vi "Main_Power.vi"() -> ()   [LabVIEW 2020]
uses:
  States.ctl
  <vilib>/Instr/_visa.llb/VISA Configure Serial Port (Serial Instr).vi
  <vilib>/Utility/file.llb/Read Delimited Spreadsheet (I64).vi
panel:
  in  "Toggle Power DAQ":bool
  out "Power":dynamicdata(graph)
  out "Last Inc Sent":string
  out "Last Speed Sent":string
  out "Next Control State":T1
  out "Next Com State":enum16{"Initialize", "Send", "Receive", "Error"}(ring)=enum."Receive"
  out "Next Cmd":enum16{"getParm", "inc", "mph", "err"}(ring)
  out "Send Buffer":string
  out "Control Error":errorcluster
  out "Com Error":errorcluster
  out "Missed Msg":u16
  out "Time Left":u32
  out "Inc Changed":bool
  out "Next MPH":u16
  out "Next Duration":u16
  out "Next Inc":u16
  out "PD READ":u8
  out "INC READ":u8
  out "MPH READ":u8
  out "dwell":u16[](array[numeric])
  out "incline":u16[](array[numeric])
  out "time":u16[](array[numeric])
  out "speed":u16[](array[numeric])
  out "input lines":i32
  in  "TestScript":path=path "C:/LabView Computer Backup SEAL2788/DonP_TRM500/FootTimeInc.txt"
  out "read buffer":string
  out "Speed Changed":bool
  in  "Manual Stop":bool
  in  "Serial Port":refnum<visa-resource-name>="COM8"
  out "FootPath":path
  out "FootPathRef":refnum<file>
  out "stopping":bool
  out "Target MPH":u16 max=12 step=1
  out "step":i32
  out "Target INC":u16 max=12 step=1
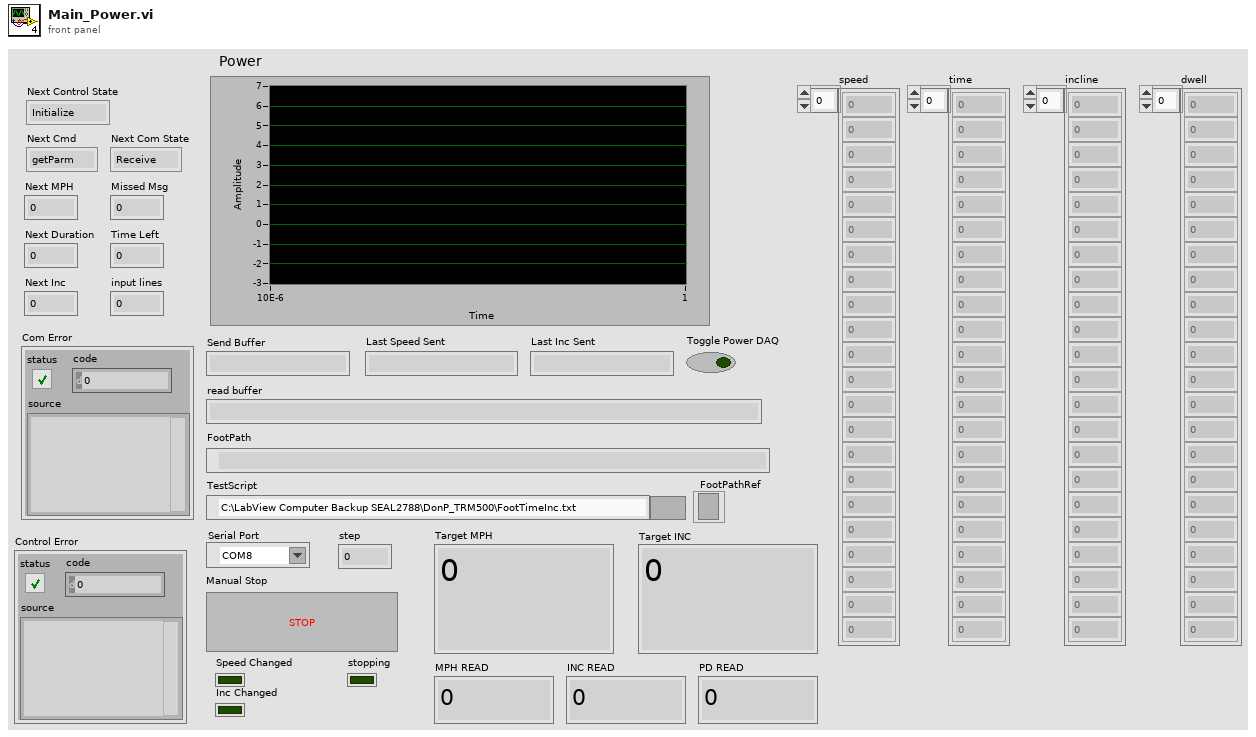
[diagram p1: front panel]
types:
  T1 = typedef "States.ctl" = enum16{"Initialize", "SetTargets", "WaitforMPH", "Dwell", "CheckTiming"}
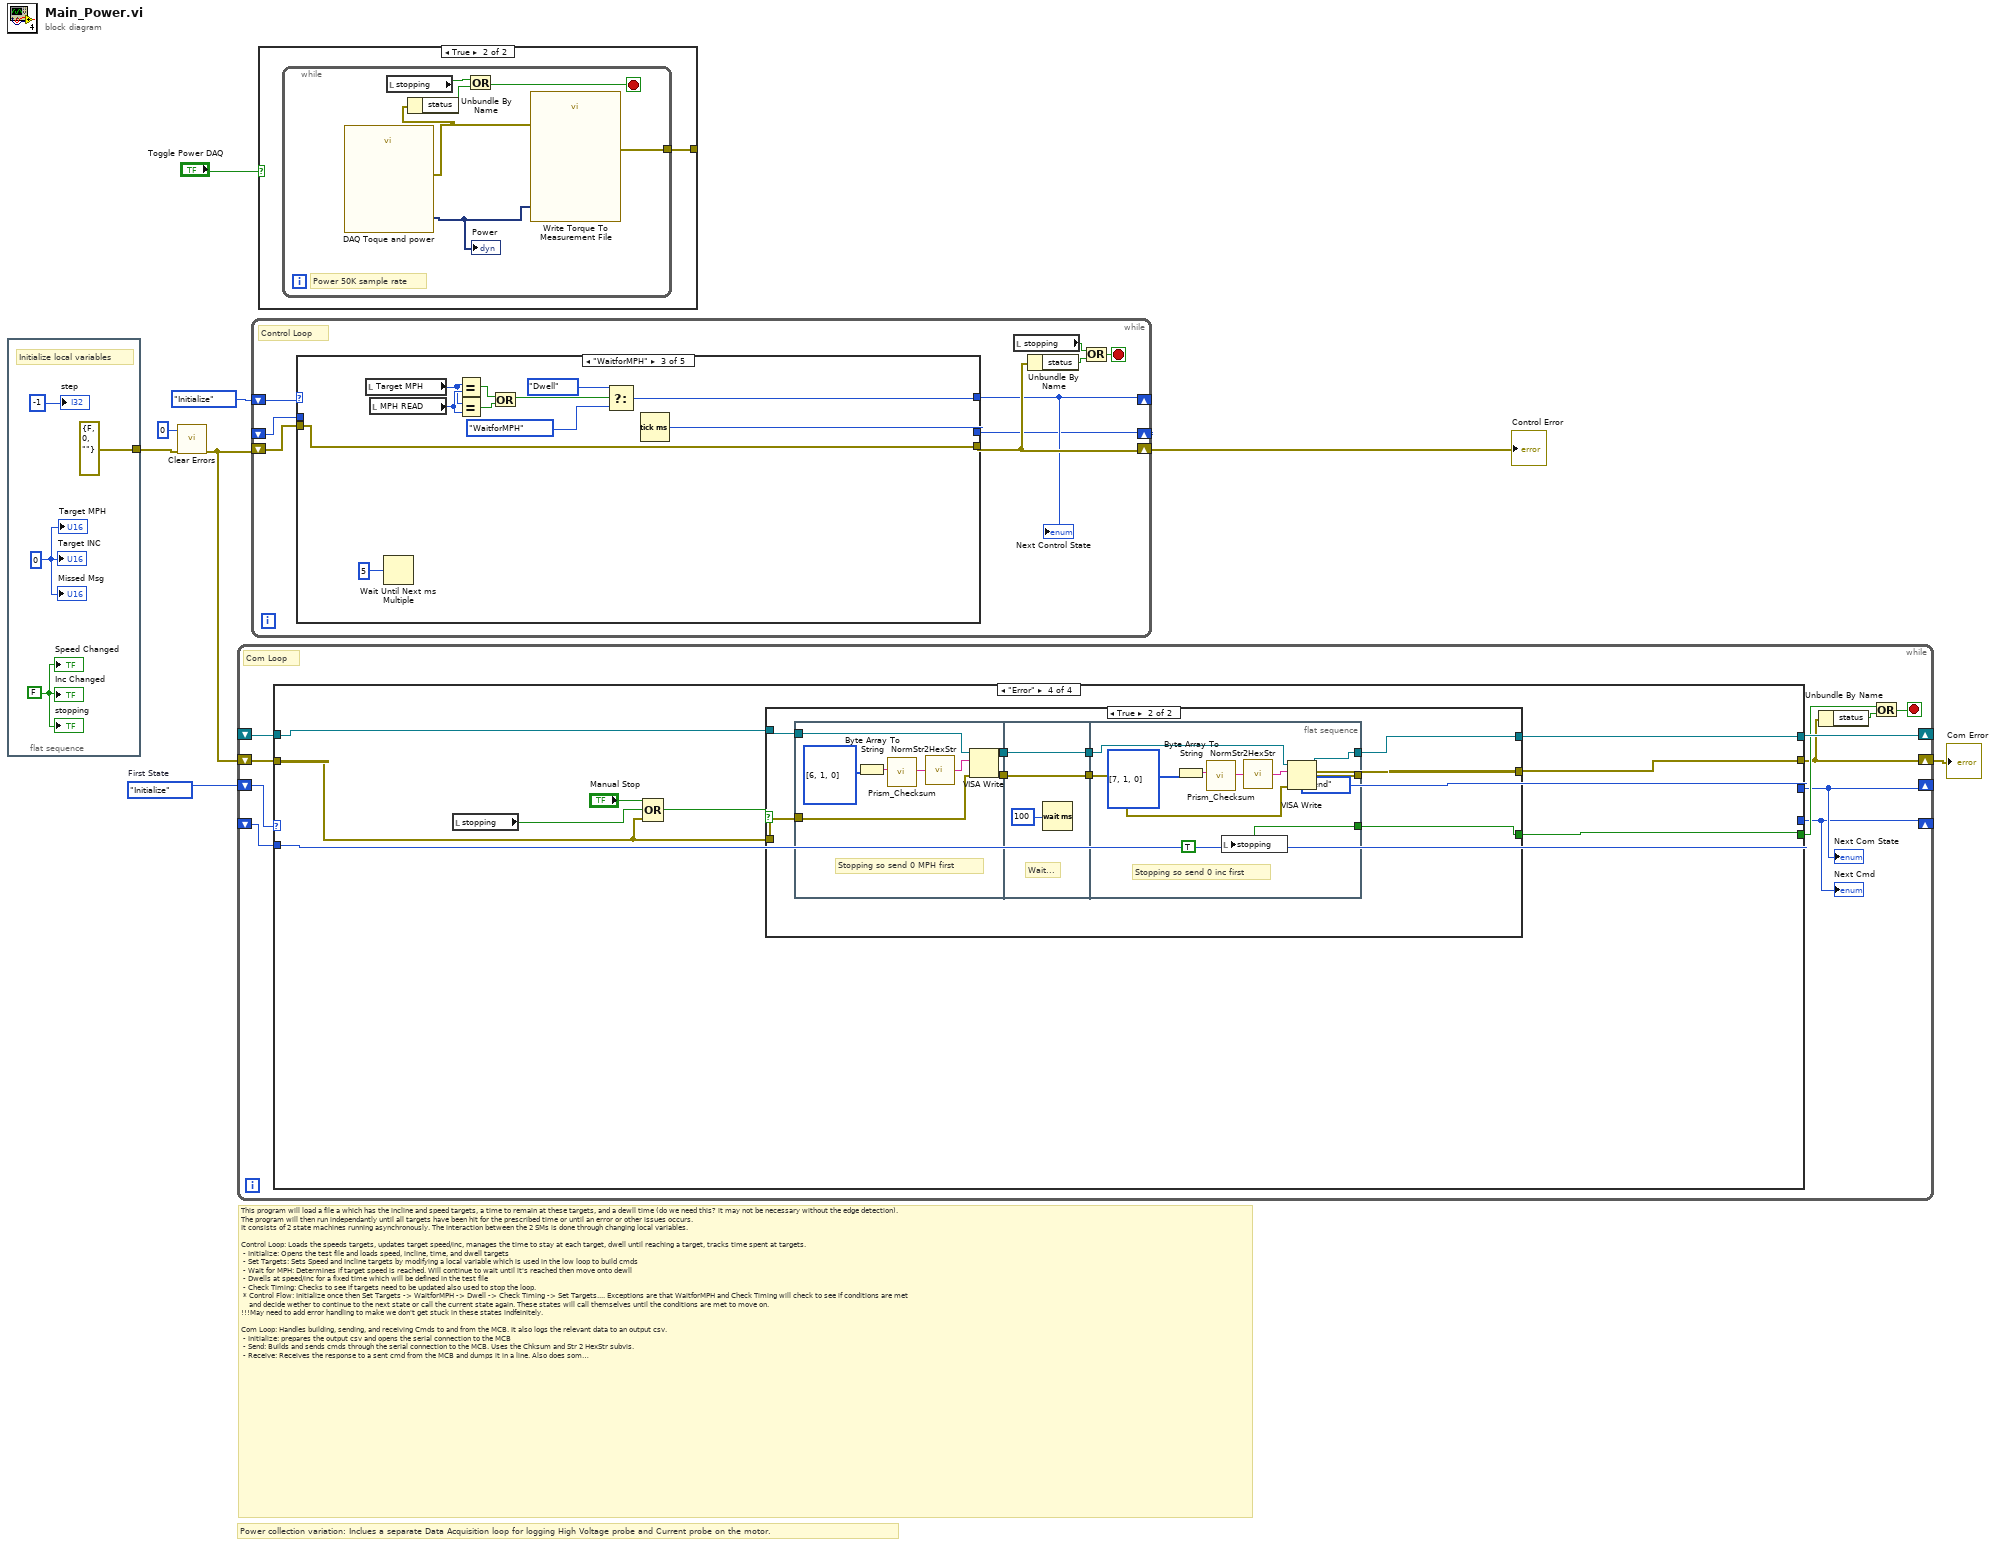
[diagram p0: block diagram]
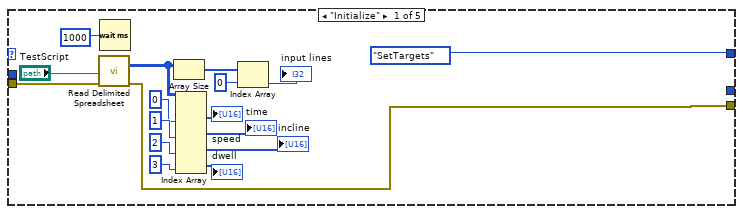
[diagram p3: hidden frame]
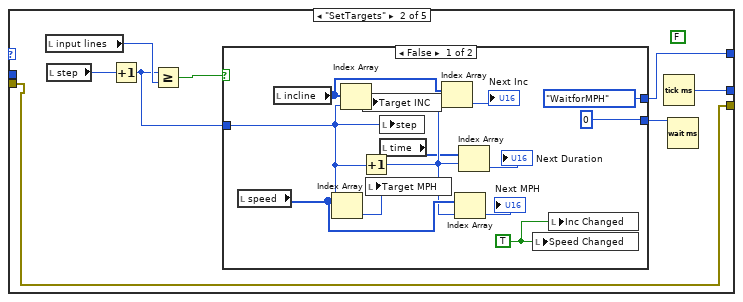
[diagram p4: hidden frame]
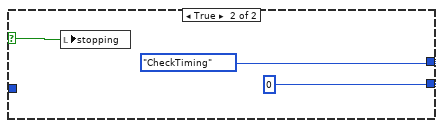
[diagram p5: hidden frame]
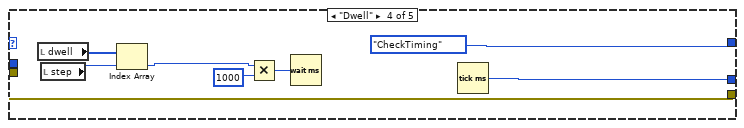
[diagram p6: hidden frame]
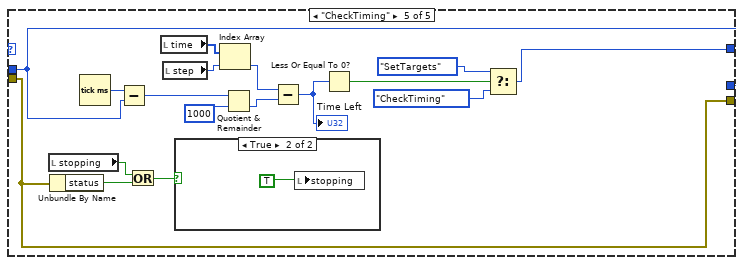
[diagram p7: hidden frame]
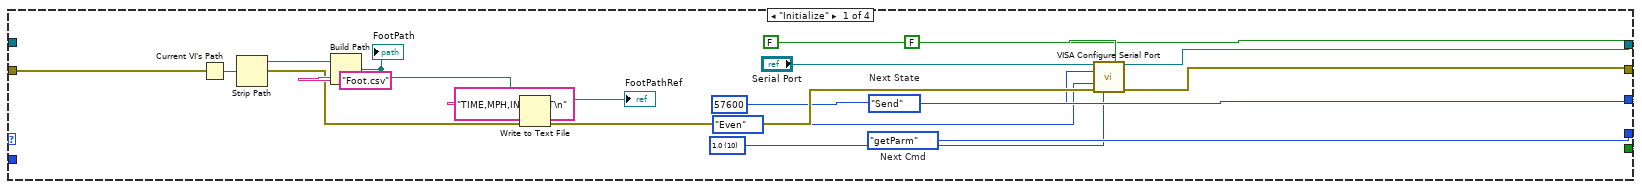
[diagram p9: hidden frame]
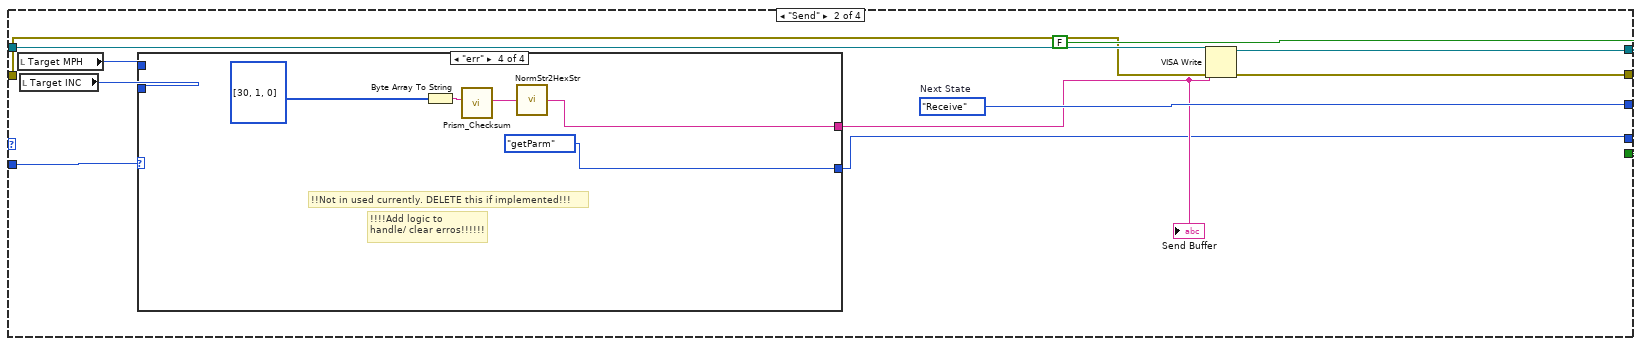
[diagram p10: hidden frame]
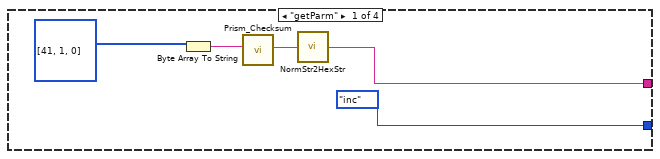
[diagram p11: hidden frame]
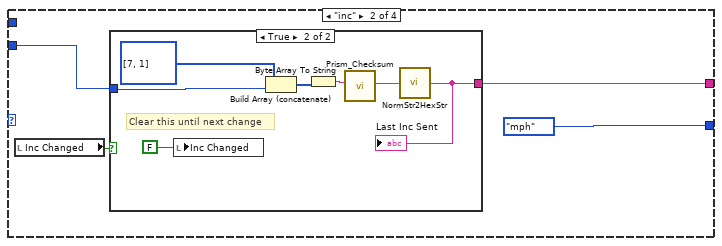
[diagram p12: hidden frame]
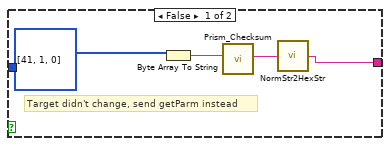
[diagram p13: hidden frame]
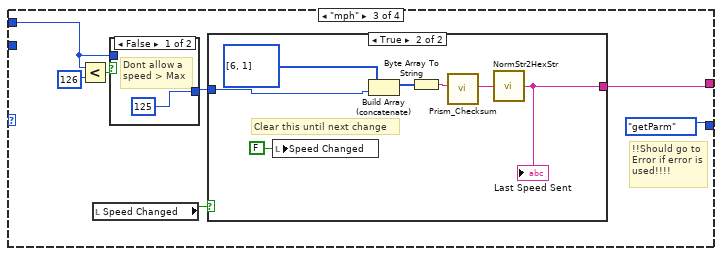
[diagram p14: hidden frame]
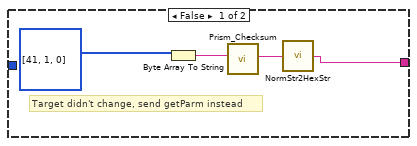
[diagram p16: hidden frame]
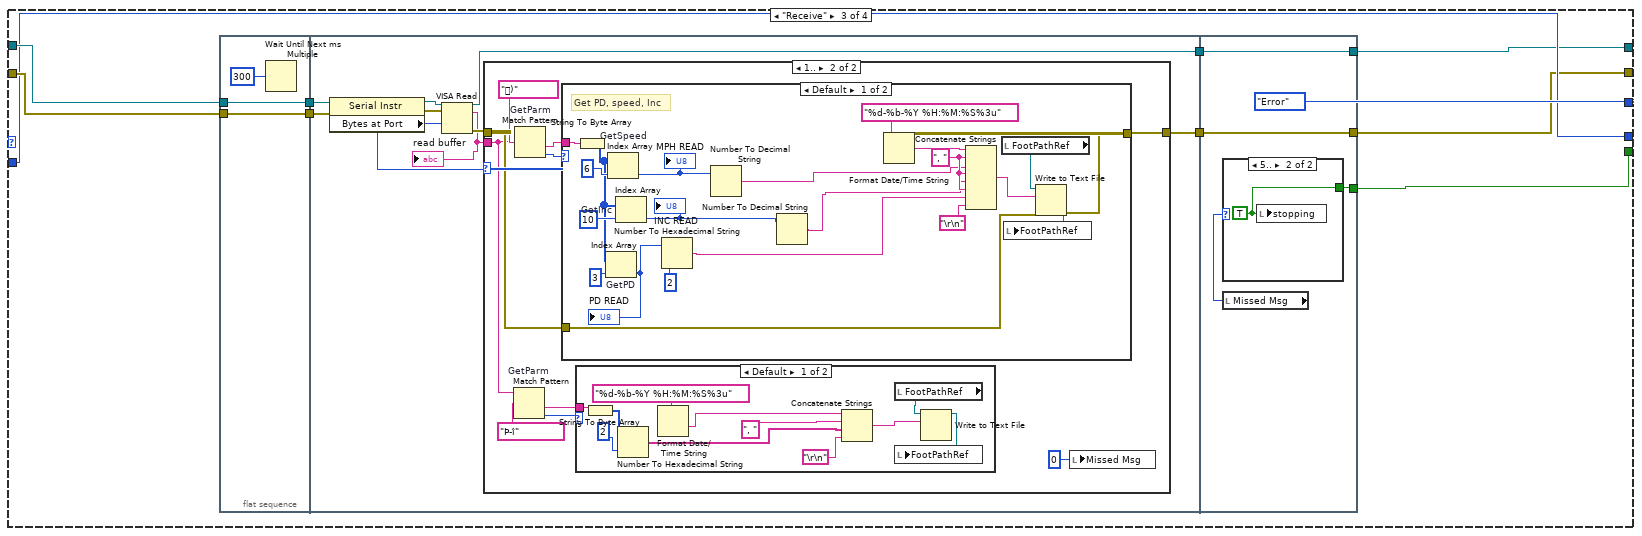
[diagram p17: hidden frame]
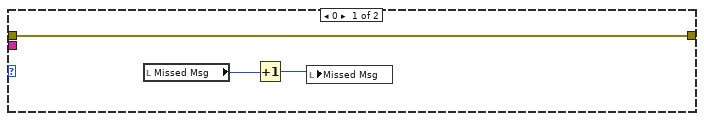
[diagram p18: hidden frame]
diagram:
  w8 = enum16{"Initialize", "Send", "Receive", "Error"}."Initialize"  # First State
  # "Power collection variation: Inclues a separate Data Acquisition loop for logging High Voltage probe and Current probe on the motor."
  # "This program will load a file a which has the incline and speed targets, a time to remain at these targets, and a dewll time (do we need this? it may not be necessary without the edge detection).\nThe program will then run independantly until all targets have been hit for the prescribed time or until an error or other issues occurs.\nIt consists of 2 state machines running asynchronously. The interaction between the 2 SMs is done through changing local variables.\n\nControl Loop: Loads the speeds targets, updates target speed/inc, manages the time to stay at each target, dwell until reaching a target, tracks time spent at targets. \n - Initialize: Opens the test file and loads speed, incline, time, and dwell targets \n - Set Targets: Sets Speed and Incline targets by modifying a local variable which is used in the low loop to build cmds \n - Wait for MPH: Determines if target speed is reached. Will continue to wait until it's reached then move onto dewll\n - Dwells at speed/inc for a fixed time which will be defined in the test file\n - Check Timing: Checks to see if targets need to be updated also used to stop the loop.\n * Control Flow: Initialize once then Set Targets -> WaitforMPH -> Dwell -> Check Timing -> Set Targets.... Exceptions are that WaitforMPH and Check Timing will check to see if conditions are met\n    and decide wether to continue to the next state or call the current state again. These states will call themselves until the conditions are met to move on. \n!!!May need to add error handling to make we don't get stuck in these states indfeinitely.\n\nCom Loop: Handles building, sending, and receiving Cmds to and from the MCB. It also logs the relevant data to an output csv.\n - Initialize: prepares the output csv and opens the serial connection to the MCB\n - Send: Builds and sends cmds through the serial connection to the MCB. Uses the Chksum and Str 2 HexStr subvis. \n - Receive: Receives the response to a sent cmd from the MCB and dumps it in a line. Also does some analysis of the response to determine current  Speed/inc/person detect\n - Error:  Stops the program. This handles labview errors and will stop the program when one is encounted. It also handles stopping when reaching the end of a test \n * Com Flow: nitialize once then Send -> Receive -> Error -> Send...\n * Send flow: GetParm -> Inc -> MPH -> GetParm etc. Exception is that it will check first to see if the target changed and if it hasn't will send getParm Instead\n!!!May need to add error handling in which case the flow should be GetParm -> MPH -> Inc -> Err -> GetParm....\n\nFiles:\n1 input file which contains the test script to run. Format: Speed, Time, Inc, Dwell. Time = time to stay at target speed/inc. Dwell = a fixed time to wait after reaching targets and before starting the Time counter. This is used to make sure the speed stablizes before starting the Time counter.\n1 output file which contains Timestamp, Speed, Incline, and a flag for if person is detected (0 = No, 1 = Yes). Format: TIME,MPH,INC,FOOT"
  n1 = flat-sequence {
    tunnel: [errorcluster {"status"=FALSE, "code"=0, "source"=""} ("error constant")] -> w4
    frame #0 {
      w10 = FALSE ("Inc Changed")
      w9 = u16 0 ("MPH")
      # "Initialize local variables"
      "stopping" <- w10
      "Target MPH" <- w9
      "step" <- -1 ("step")
      "Target INC" <- w9
      "Speed Changed" <- w10
      "Inc Changed" <- w10
      "Missed Msg" <- w9
    }
  }
  n2 = call <vilib>:"Clear Errors.vi"("error in (no error)"=w4, "specific error code to clear (0: all)"=0) -> ("error out"=w3:errorcluster)  [unwired: 4 in, 1 out]
  n3 = while {
    shift-right: [w17] -> w7
    shift-left: w3 -> [w23]
    shift-right: [w20] -> _
    shift-left: _ -> [w22]
    shift-right: [w14] -> _
    shift-left: w8 -> [w21]
    shift-right: [w13] -> _
    shift-left: _ -> [w19]
    stop <- w16 stop-if-true
    # "Com Loop"
    n4 = case shown="\"Error\"" w21 {
      tunnel: w23 -> [w29 w43 w106 w176]
      tunnel: w22 -> [_ w50 w108 w174]
      tunnel: [w39 w52 w102 w173] -> w20
      tunnel: [w38 w51 w101 w175] -> w17
      tunnel: [w35 w46 enum16{"Initialize", "Send", "Receive", "Error"}."Error" enum16{"Initialize", "Send", "Receive", "Error"}."Send"] -> w14
      tunnel: [w37 w44 w105 w181] -> w13
      tunnel: w19 -> [_ w42 w105 w181]
      tunnel: [FALSE FALSE w98 w177] -> w18
      frame "Initialize" {
        w24 = u16 10 items=["1.0"=10, "1.5"=15, "2.0"=20] ("stop bits (10: 1 bit)")
        w35 = enum16{"Initialize", "Send", "Receive", "Error"}."Send"  # Next State
        w37 = enum16{"getParm", "inc", "mph", "err"}."getParm"  # Next Cmd
        n5 = Current VI's Path() -> (path=w34:path)
        n6 = Strip Path(path=w34) -> (stripped path=w33:path)  [unwired: 1 out]
        n7 = Build Path(base path=w33, name or relative path="Foot.csv") -> (appended path=w30:path)
        "FootPath" <- w30
        n8 = Write to Text File(file (use dialog)=w30, text="TIME,MPH,INC,FOOT\n", error in=w29) -> (refnum out=→"FootPathRef":refnum<file>, error out=w28:errorcluster)  [unwired: 1 in, 1 out]
        n9 = call-poly "VISA Configure Serial Port"("VISA resource name"="Serial Port", "Enable Termination\nChar (T)"=FALSE ("Enable Termination\nChar (T)"), "baud rate (9600)"=u32 57600, "parity (0:none)"=enum16{"None", "Odd", "Even", "Mark", "Space"}."Even", "error in (no error)"=w28, "stop bits (10: 1 bit)"=w24) -> ("VISA resource name out"=w39:refnum<visa-resource-name>, "error out"=w38:errorcluster)  [unwired: 8 in]
      }
      frame "Send" {
        w46 = enum16{"Initialize", "Send", "Receive", "Error"}."Receive"  # Next State
        n10 = local read "Target MPH"() -> (w48:u16)
        n11 = local read "Target INC"() -> (w47:u16)
        n12 = case shown="\"err\"" w42 {
          tunnel: w48 -> [_ _ w74 _]
          tunnel: w47 -> [_ w61 _ _]
          tunnel: [w53 w60 w78 w94] -> w45
          tunnel: [enum16{"getParm", "inc", "mph", "err"}."inc" enum16{"getParm", "inc", "mph", "err"}."mph" enum16{"getParm", "inc", "mph", "err"}."getParm" enum16{"getParm", "inc", "mph", "err"}."getParm"] -> w44
          frame "getParm" {
            n13 = Byte Array To String(unsigned byte array=u8[] [41, 1, 0]) -> (string=w55:string)
            n14 = call "Prism_Checksum.vi"("ID +DB+ Data"=w55) -> ("Full Cmd"=w54:string)  [unwired: 10 in]
            n15 = call "NormStr2HexStr.vi"("string"=w54) -> ("hex string"=w53:string)
          }
          frame "inc" {
            n16 = local read "Inc Changed"() -> (w58:bool)
            n17 = case shown="True" w58 {
              tunnel: w61 -> [_ w69]
              tunnel: [w62 w67] -> w60
              frame False {
                # "Target didn't change, send getParm instead"
                n18 = Byte Array To String(unsigned byte array=u8[] [41, 1, 0]) -> (string=w64:string)
                n19 = call "Prism_Checksum.vi"("ID +DB+ Data"=w64) -> ("Full Cmd"=w63:string)  [unwired: 10 in]
                n20 = call "NormStr2HexStr.vi"("string"=w63) -> ("hex string"=w62:string)
              }
              frame True {
                # "Clear this until next change"
                n21 = local write "Inc Changed"(FALSE ("Value Changed")) -> ()
                n22 = Build Array (concatenate)(u8[] [7, 1] ("unsigned byte array"), w69) -> (w68:u16[])
                n23 = Byte Array To String(unsigned byte array=w68) -> (string=w71:string)
                n24 = call "Prism_Checksum.vi"("ID +DB+ Data"=w71) -> ("Full Cmd"=w72:string)  [unwired: 10 in]
                n25 = call "NormStr2HexStr.vi"("string"=w72) -> ("hex string"=w67:string)
                "Last Inc Sent" <- w67
              }
            }
          }
          frame "mph" {
            # "!!Should go to\nError if error is\nused!!!!"
            n26 = Less?(x=w74, y=u16 126) -> (x < y?=w76:bool)
            n27 = local read "Speed Changed"() -> (w77:bool)
            n28 = case shown="False" w76 {
              tunnel: w74 -> [_ w81]
              tunnel: [u16 125 ("Target MPH") w81] -> w73
              frame False {
                # "Dont allow a\nspeed > Max"
              }
              frame True {
              }
            }
            n29 = case shown="True" w77 {
              tunnel: [w82 w89] -> w78
              tunnel: w73 -> [_ w87]
              frame False {
                # "Target didn't change, send getParm instead"
                n30 = Byte Array To String(unsigned byte array=u8[] [41, 1, 0]) -> (string=w84:string)
                n31 = call "Prism_Checksum.vi"("ID +DB+ Data"=w84) -> ("Full Cmd"=w83:string)  [unwired: 10 in]
                n32 = call "NormStr2HexStr.vi"("string"=w83) -> ("hex string"=w82:string)
              }
              frame True {
                # "Clear this until next change"
                n33 = local write "Speed Changed"(FALSE ("Value Changed")) -> ()
                n34 = Build Array (concatenate)(u8[] [6, 1] ("unsigned byte array"), w87) -> (w88:u16[])
                n35 = Byte Array To String(unsigned byte array=w88) -> (string=w91:string)
                n36 = call "Prism_Checksum.vi"("ID +DB+ Data"=w91) -> ("Full Cmd"=w92:string)  [unwired: 10 in]
                n37 = call "NormStr2HexStr.vi"("string"=w92) -> ("hex string"=w89:string)
                "Last Speed Sent" <- w89
              }
            }
          }
          frame "err" {
            # "!!Not in used currently. DELETE this if implemented!!!"
            # "!!!!Add logic to\nhandle/ clear erros!!!!!!"
            n38 = Byte Array To String(unsigned byte array=u8[] [30, 1, 0]) -> (string=w96:string)
            n39 = call "Prism_Checksum.vi"("ID +DB+ Data"=w96) -> ("Full Cmd"=w97:string)  [unwired: 10 in]
            n40 = call "NormStr2HexStr.vi"("string"=w97) -> ("hex string"=w94:string)
          }
        }
        "Send Buffer" <- w45
        n41 = VISA Write(VISA resource name=w50, write buffer=w45, error in (no error)=w43) -> (VISA resource name out=w52:refnum<visa-resource-name>, error out=w51:errorcluster)  [unwired: 1 out]
      }
      frame "Receive" {
        n42 = flat-sequence {
          tunnel: w108 -> [w110]
          tunnel: w106 -> [w109]
          tunnel: [w110] -> w104
          tunnel: [w109] -> w103
          tunnel: w104 -> [w120]
          tunnel: w103 -> [w119]
          tunnel: [w112] -> w100
          tunnel: [w116] -> w99
          tunnel: [w169] -> w101
          tunnel: [w170] -> w102
          tunnel: w100 -> [w170]
          tunnel: w99 -> [w169]
          tunnel: [w167] -> w98
          frame #0 {
            n43 = Wait Until Next ms Multiple(millisecond multiple=u32 300) -> ()  [unwired: 1 out]
          }
          frame #1 {
            n44 = property class="Serial Instr"(reference=w120, error in=w119) -> (reference out=w117:refnum<visa-resource-name>, error out=w118:errorcluster, "Bytes at Port"=w115:u32)
            n45 = VISA Read(VISA resource name=w117, byte count=w115, error in (no error)=w118) -> (VISA resource name out=w112:refnum<visa-resource-name>, read buffer=w113:string, error out=w114:errorcluster)  [unwired: 1 out]
            "read buffer" <- w113
            n46 = case shown="1.." w115 {
              tunnel: [w123 w130] -> w116
              tunnel: w114 -> [w123 w129]
              tunnel: w113 -> [_ w128]
              frame 0 {
                n47 = local read "Missed Msg"() -> (w122:u16)
                n48 = Increment(x=w122) -> (x+1=w121:u16)
                n49 = local write "Missed Msg"(w121) -> ()
              }
              frame 1.. {
                n50 = Match Pattern "GetParm"(string=w128, regular expression="Þ­î") -> (after substring=w125:string, offset past match=w126:i32)  [unwired: 1 in, 2 out]
                n51 = Match Pattern "GetParm"(string=w128, regular expression="ޭ)") -> (after substring=w132:string, offset past match=w131:i32)  [unwired: 1 in, 2 out]
                n52 = case shown="Default" w131 {
                  tunnel: w132 -> [w146 _]
                  tunnel: [w159 w166] -> w130
                  tunnel: w129 -> [w154 w166]
                  frame Default {
                    w153 = ", "
                    # "Get PD, speed, Inc"
                    n53 = String To Byte Array(string=w146) -> (unsigned byte array=w162:u8[])
                    n54 = Index Array "GetPD"(array=w162, index=3) -> (element=w156:u8)
                    "PD READ" <- w156
                    n55 = Index Array "GetSpeed"(array=w162, index=6) -> (element=w148:u8)
                    "MPH READ" <- w148
                    n56 = Index Array "GetInc"(array=w162, index=10) -> (element=w147:u8)
                    "INC READ" <- w147
                    n57 = Number To Hexadecimal String(1:i16 2 ("width (-)"), 2:w156) -> (0:w151:string)
                    n58 = Number To Decimal String(number=w148) -> (decimal integer string=w150:string)  [unwired: 1 in]
                    n59 = Number To Decimal String(number=w147) -> (decimal integer string=w149:string)  [unwired: 1 in]
                    n60 = Format Date/Time String(time format string (%c)="%d-%b-%Y %H:%M:%S%3u") -> (date/time string=w157:string)  [unwired: 2 in]
                    n61 = Concatenate Strings(w157, w153, w150, w153, w149, w153, w151, "\r\n") -> (w160:string)
                    n62 = local read "FootPathRef"() -> (w158:refnum<file>)
                    n63 = Write to Text File(file (use dialog)=w158, text=w160, error in=w154) -> (refnum out=w152:refnum<file>, error out=w159:errorcluster)  [unwired: 1 in, 1 out]
                    n64 = local write "FootPathRef"(w152) -> ()
                  }
                  frame -1 {
                  }
                }
                n65 = case shown="Default" w126 {
                  tunnel: w125 -> [w139 _]
                  frame Default {
                    n66 = String To Byte Array(string=w139) -> (unsigned byte array=w137:u8[])
                    n67 = Number To Hexadecimal String(1:i16 2 ("width (-)"), 2:w137) -> (0:w134:string[])
                    n68 = Format Date/Time String(time format string (%c)="%d-%b-%Y %H:%M:%S%3u") -> (date/time string=w141:string)  [unwired: 2 in]
                    n69 = Concatenate Strings(w141, ", ", w134, "\r\n") -> (w140:string)
                    n70 = local read "FootPathRef"() -> (w144:refnum<file>)
                    n71 = Write to Text File(file (use dialog)=w144, text=w140) -> (refnum out=w143:refnum<file>)  [unwired: 2 in, 2 out]
                    n72 = local write "FootPathRef"(w143) -> ()
                  }
                  frame -1 {
                  }
                }
                n73 = local write "Missed Msg"(u16 0 ("Missed Msg")) -> ()
              }
            }
          }
          frame #2 {
            n74 = local read "Missed Msg"() -> (w168:u16)
            n75 = case shown="5.." w168 {
              tunnel: [FALSE ("stopping") w172] -> w167
              frame ..4 {
              }
              frame 5.. {
                w172 = TRUE ("stopping")
                n76 = local write "stopping"(w172) -> ()
              }
            }
          }
        }
      }
      frame "Error" {
        n77 = local read "stopping"() -> (w178:bool)
        n78 = Compound Arithmetic op=OR("Manual Stop", w178, w176) -> (w180:bool)
        n79 = case shown="True" w180 {
          tunnel: [FALSE w186] -> w177
          tunnel: w176 -> [w184 w194]
          tunnel: [w184 w193] -> w175
          tunnel: w174 -> [w183 w192]
          tunnel: [w183 w191] -> w173
          frame False {
          }
          frame True {
            n80 = flat-sequence {
              tunnel: w194 -> [w198]
              tunnel: w192 -> [w196]
              tunnel: [w197] -> w190
              tunnel: [w195] -> w189
              tunnel: w190 -> [w205]
              tunnel: w189 -> [w204]
              tunnel: [w205] -> w188
              tunnel: [w204] -> w187
              tunnel: [w207] -> w191
              tunnel: [w206] -> w193
              tunnel: w188 -> [w208]
              tunnel: w187 -> [w209]
              tunnel: [w214] -> w186
              frame #0 {
                # "Stopping so send 0 MPH first"
                n81 = Byte Array To String(unsigned byte array=u8[] [6, 1, 0]) -> (string=w202:string)
                n82 = call "Prism_Checksum.vi"("ID +DB+ Data"=w202) -> ("Full Cmd"=w201:string)  [unwired: 10 in]
                n83 = call "NormStr2HexStr.vi"("string"=w201) -> ("hex string"=w200:string)
                n84 = VISA Write(VISA resource name=w196, write buffer=w200, error in (no error)=w198) -> (VISA resource name out=w195:refnum<visa-resource-name>, error out=w197:errorcluster)  [unwired: 1 out]
              }
              frame #1 {
                # "Wait..."
                n85 = Wait (ms)(milliseconds to wait=u32 100) -> ()  [unwired: 1 out]
              }
              frame #2 {
                w214 = TRUE ("stopping")
                # "Stopping so send 0 inc first"
                n86 = Byte Array To String(unsigned byte array=u8[] [7, 1, 0]) -> (string=w213:string)
                n87 = call "Prism_Checksum.vi"("ID +DB+ Data"=w213) -> ("Full Cmd"=w212:string)  [unwired: 10 in]
                n88 = local write "stopping"(w214) -> ()
                n89 = call "NormStr2HexStr.vi"("string"=w212) -> ("hex string"=w211:string)
                n90 = VISA Write(VISA resource name=w209, write buffer=w211, error in (no error)=w208) -> (VISA resource name out=w207:refnum<visa-resource-name>, error out=w206:errorcluster)  [unwired: 1 out]
              }
            }
          }
        }
      }
    }
    "Next Com State" <- w14
    "Next Cmd" <- w13
    n91 = Unbundle By Name(w17) -> ("status"=w15:bool)
    n92 = Or(x=w18, y=w15) -> (x .or. y?=w16:bool)
  }
  "Com Error" <- w7
  n93 = while {
    shift-right: [w220] -> w6
    shift-left: w3 -> [w223]
    shift-right: [w218] -> _
    shift-left: _ -> [w217]
    shift-right: [w219] -> _
    shift-left: States."Initialize" ("First State") -> [w216]
    stop <- w221 stop-if-true
    # "Control Loop"
    n94 = case shown="\"WaitforMPH\"" w216 {
      tunnel: w223 -> [w238 w241 w274 w280 w284]
      tunnel: [w228 w241 w274 w280 w284] -> w220
      tunnel: [States."SetTargets" ("First State") w245 w272 States."CheckTiming" ("First State") w285] -> w219
      tunnel: [_ w243 w273 w277 w296] -> w218
      tunnel: w217 -> [_ _ _ _ w296]
      frame "Initialize" {
        n95 = call-poly <vilib>:"Read Delimited Spreadsheet.vi"("file path (dialog if empty)"="TestScript", "error in (no error)"=w238) -> ("all rows"=w234:i64[][], "error out"=w228:errorcluster)  [unwired: 8 in, 4 out]
        n96 = Wait (ms)(milliseconds to wait=u32 1000) -> ()  [unwired: 1 out]
        n97 = Array Size(array=w234) -> (size(s)=w236:i32[])
        n98 = Index Array(array=w234, index (col) #1=0 ("index"), index (col) #2=1 ("index (col)"), index (col) #3=2 ("index (col)"), index (col) #4=3 ("index (col)")) -> (element #1=→"speed":i64[], element #2=→"time":i64[], element #3=→"incline":i64[], element #4=→"dwell":i64[])  [unwired: 4 in]
        n99 = Index Array(array=w236, index=0) -> (element=→"input lines":i32)
      }
      frame "SetTargets" {
        (unwired) FALSE
        n100 = local read "input lines"() -> (w247:i32)
        n101 = local read "step"() -> (w248:i32)
        n102 = Increment(x=w248) -> (x+1=w242:i32)
        n103 = Greater Or Equal?(x=w242, y=w247) -> (x >= y?=w246:bool)
        n104 = case shown="False" w246 {
          selector: w246 -> [_ w264]
          tunnel: [States."WaitforMPH" ("First State") States."CheckTiming" ("First State")] -> w245
          tunnel: [u32 0 ("milliseconds to wait") u32 0 ("milliseconds to wait")] -> w244
          tunnel: w242 -> [w259 _]
          frame False {
            w250 = TRUE ("Value Changed")
            n105 = local read "speed"() -> (w258:u16[])
            n106 = local read "incline"() -> (w257:u16[])
            n107 = Index Array(array=w258, index=w259) -> (element=w261:u16)
            n108 = Index Array(array=w257, index=w259) -> (element=w260:u16)
            n109 = Increment(x=w259) -> (x+1=w256:i32)
            n110 = local write "Target INC"(w260) -> ()
            n111 = local write "Target MPH"(w261) -> ()
            n112 = local write "step"(w259) -> ()
            n113 = local read "time"() -> (w255:u16[])
            n114 = Index Array(array=w257, index=w256) -> (element=→"Next Inc":u16)
            n115 = Index Array(array=w258, index=w256) -> (element=→"Next MPH":u16)
            n116 = Index Array(array=w255, index=w256) -> (element=→"Next Duration":u16)
            n117 = local write "Speed Changed"(w250) -> ()
            n118 = local write "Inc Changed"(w250) -> ()
          }
          frame True {
            n119 = local write "stopping"(w264) -> ()
          }
        }
        n120 = Tick Count (ms)() -> (millisecond timer value=w243:u32)
        n121 = Wait (ms)(milliseconds to wait=w244) -> ()  [unwired: 1 out]
      }
      frame "WaitforMPH" {
        n122 = local read "Target MPH"() -> (w267:u16)
        n123 = local read "MPH READ"() -> (w268:u8)
        n124 = Wait Until Next ms Multiple(millisecond multiple=u32 5) -> ()  [unwired: 1 out]
        n125 = Equal?(x=w267, y=w268) -> (x = y?=w270:bool)
        n126 = Equal?(x=w267, y=w268) -> (x = y?=w269:bool)
        n127 = Or(x=w270, y=w269) -> (x .or. y?=w271:bool)
        n128 = Select(t=States."Dwell" ("First State"), s=w271, f=States."WaitforMPH" ("First State")) -> (s? t:f=w272:T1)
        n129 = Tick Count (ms)() -> (millisecond timer value=w273:u32)
      }
      frame "Dwell" {
        n130 = local read "dwell"() -> (w278:u16[])
        n131 = local read "step"() -> (w279:i32)
        n132 = Index Array(array=w278, index=w279) -> (element=w283:u16)
        n133 = Multiply(x=w283, y=u16 1000) -> (x*y=w281:u16)
        n134 = Wait (ms)(milliseconds to wait=w281) -> ()  [unwired: 1 out]
        n135 = Tick Count (ms)() -> (millisecond timer value=w277:u32)
      }
      frame "CheckTiming" {
        n136 = local read "stopping"() -> (w298:bool)
        n137 = Unbundle By Name(w284) -> ("status"=w299:bool)
        n138 = Tick Count (ms)() -> (millisecond timer value=w300:u32)
        n139 = Subtract(x=w300, y=w296) -> (x-y=w295:u32)
        n140 = Or(x=w298, y=w299) -> (x .or. y?=w297:bool)
        n141 = local read "time"() -> (w293:u16[])
        n142 = local read "step"() -> (w292:i32)
        n143 = case shown="True" w297 {
          frame False {
          }
          frame True {
            n144 = local write "stopping"(TRUE ("stopping")) -> ()
          }
        }
        n145 = Index Array(array=w293, index=w292) -> (element=w290:u16)
        n146 = Quotient & Remainder(x=w295, y=u32 1000) -> (floor(x/y)=w291:u32)  [unwired: 1 out]
        n147 = Subtract(x=w290, y=w291) -> (x-y=w289:u32)
        "Time Left" <- w289
        n148 = Less Or Equal To 0?(x=w289) -> (x <= 0?=w288:bool)
        n149 = Select(t=States."SetTargets" ("First State"), s=w288, f=States."CheckTiming" ("First State")) -> (s? t:f=w285:T1)
      }
    }
    "Next Control State" <- w219
    n150 = local read "stopping"() -> (w215:bool)
    n151 = Unbundle By Name(w220) -> ("status"=w222:bool)
    n152 = Or(x=w215, y=w222) -> (x .or. y?=w221:bool)
  }
  "Control Error" <- w6
  n153 = case shown="True" "Toggle Power DAQ" {
    tunnel: [_ w302] -> _
    frame False {
    }
    frame True {
      n154 = while {
        tunnel: [w305] -> w302
        stop <- w307 stop-if-true
        # "Power 50K sample rate"
        n155 = call "DAQ Toque and power"() -> ("data"=w303:dynamicdata, "error out"=w306:errorcluster)  [unwired: 16 in, 2 out]
        "Power" <- w303
        n156 = local read "stopping"() -> (w304:bool)
        n157 = Unbundle By Name(w306) -> ("status"=w308:bool)
        n158 = Or(x=w304, y=w308) -> (x .or. y?=w307:bool)
        n159 = call "Write Torque To Measurement File"("Signals"=w303, "error in (no error)"=w306) -> ("error out"=w305:errorcluster)  [unwired: 15 in, 2 out]
      }
    }
  }
